vi "Calculate Trapazoidal Profile.vi"(4 "t":dbl, 5 "Max Velocity":dbl, 6 "Final Position":dbl, 7 "Max Acceleration":dbl, 9 "Final Velocity":dbl, 10 "Initial Position":dbl, 11 "Initial Velocity":dbl) -> (2 "Result Position":dbl, 3 "Result Velocity":dbl)   [LabVIEW 2019]
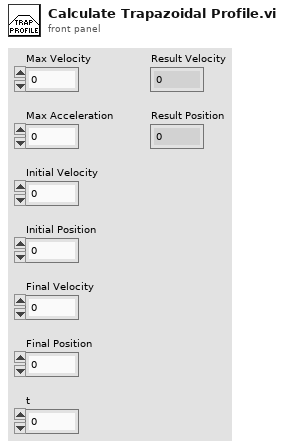
[diagram p1: front panel]
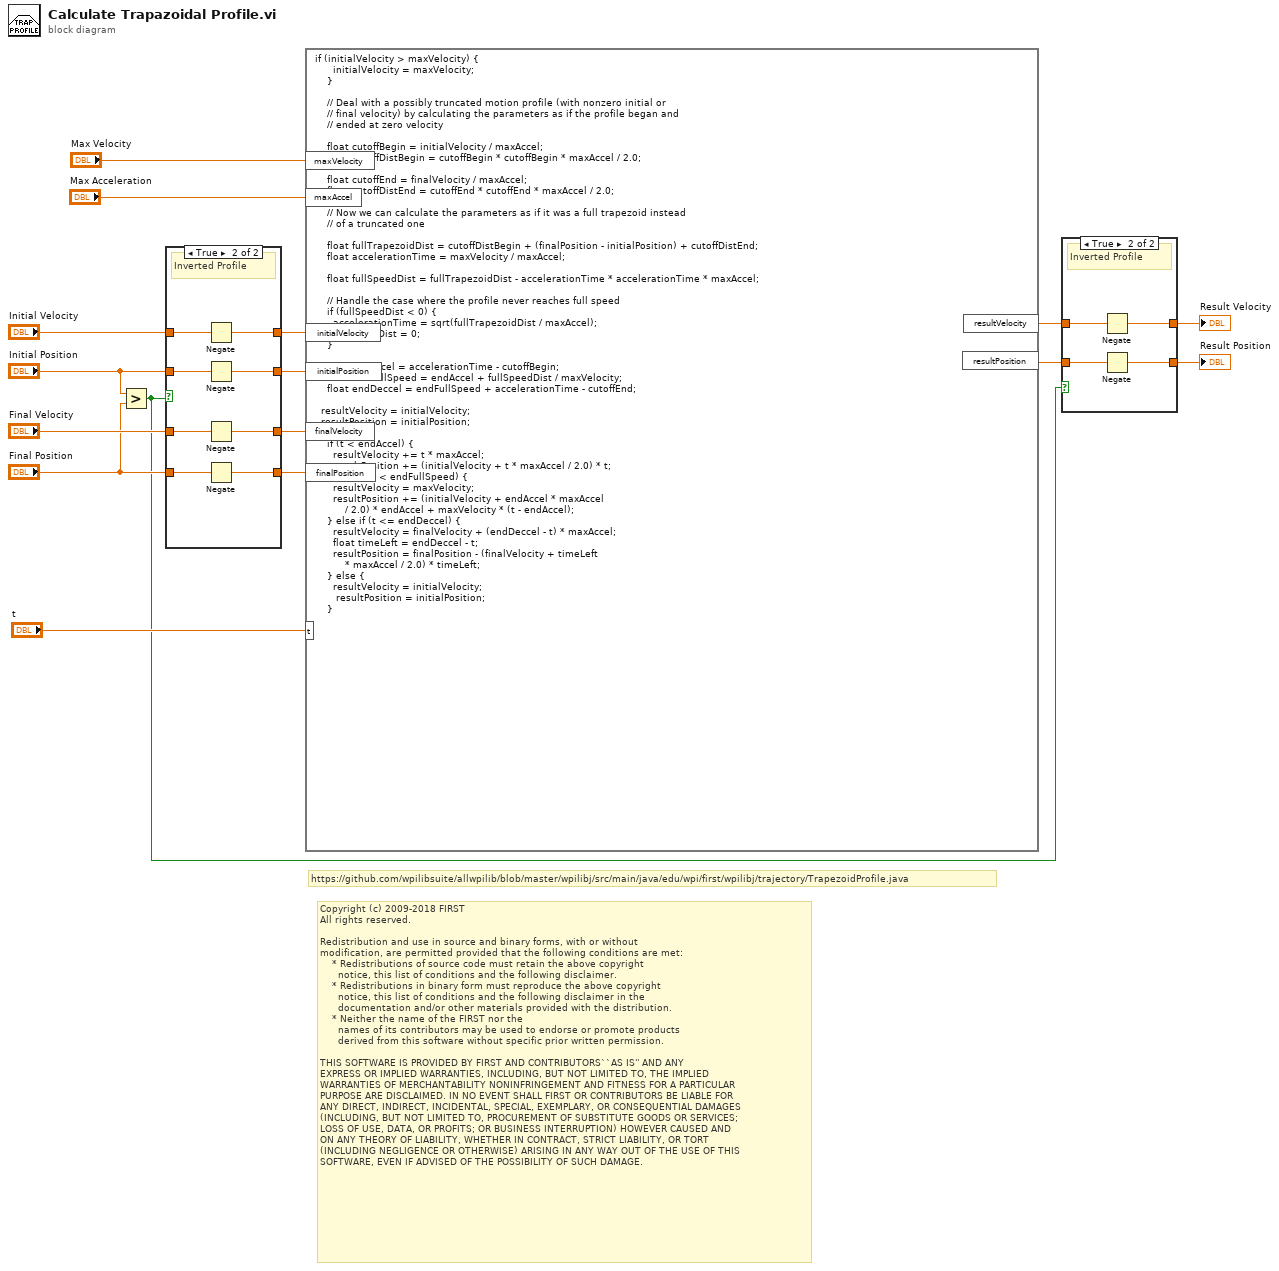
[diagram p0: block diagram]
diagram:
  # "Copyright (c) 2009-2018 FIRST\nAll rights reserved.\n\nRedistribution and use in source and binary forms, with or without\nmodification, are permitted provided that the following conditions are met:\n    * Redistributions of source code must retain the above copyright\n      notice, this list of conditions and the following disclaimer.\n    * Redistributions in binary form must reproduce the above copyright\n      notice, this list of conditions and the following disclaimer in the\n      documentation and/or other materials provided with the distribution.\n    * Neither the name of the FIRST nor the\n      names of its contributors may be used to endorse or promote products\n      derived from this software without specific prior written permission.\n\nTHIS SOFTWARE IS PROVIDED BY FIRST AND CONTRIBUTORS``AS IS'' AND ANY\nEXPRESS OR IMPLIED WARRANTIES, INCLUDING, BUT NOT LIMITED TO, THE IMPLIED\nWARRANTIES OF MERCHANTABILITY NONINFRINGEMENT AND FITNESS FOR A PARTICULAR\nPURPOSE ARE DISCLAIMED. IN NO EVENT SHALL FIRST OR CONTRIBUTORS BE LIABLE FOR\nANY DIRECT, INDIRECT, INCIDENTAL, SPECIAL, EXEMPLARY, OR CONSEQUENTIAL DAMAGES\n(INCLUDING, BUT NOT LIMITED TO, PROCUREMENT OF SUBSTITUTE GOODS OR SERVICES;\nLOSS OF USE, DATA, OR PROFITS; OR BUSINESS INTERRUPTION) HOWEVER CAUSED AND\nON ANY THEORY OF LIABILITY, WHETHER IN CONTRACT, STRICT LIABILITY, OR TORT\n(INCLUDING NEGLIGENCE OR OTHERWISE) ARISING IN ANY WAY OUT OF THE USE OF THIS\nSOFTWARE, EVEN IF ADVISED OF THE POSSIBILITY OF SUCH DAMAGE."
  # "https://github.com/wpilibsuite/allwpilib/blob/master/wpilibj/src/main/java/edu/wpi/first/wpilibj/trajectory/TrapezoidProfile.java"
  n1 = Greater?(x="Initial Position", y="Final Position") -> (0:w1:bool)
  n2 = case shown="True" w1 {
    tunnel: "Final Velocity" -> [w18 w28]
    tunnel: [w18 w27] -> w12
    tunnel: "Final Position" -> [w17 w26]
    tunnel: [w17 w25] -> w10
    tunnel: "Initial Position" -> [w19 w24]
    tunnel: [w19 w23] -> w8
    tunnel: "Initial Velocity" -> [w20 w22]
    tunnel: [w20 w21] -> w6
    frame False {
    }
    frame True {
      # "Inverted Profile"
      n3 = Negate(x=w22) -> (-x=w21:dbl)
      n4 = Negate(x=w24) -> (-x=w23:dbl)
      n5 = Negate(x=w28) -> (-x=w27:dbl)
      n6 = Negate(x=w26) -> (-x=w25:dbl)
    }
  }
  n7 = formula code="if (initialVelocity > maxVelocity) {\n      initialVelocity = maxVelocity;\n    }\n\n    // Deal with a possibly truncated motion profile (with nonzero initial or\n    // final velocity) by calculating the parameters as if the profile began and\n    // ended at zero velocity\n\n    float cutoffBegin = initialVelocity / maxAccel;\n    float cutoffDistBegin = cutoffBegin * cutoffBegin * maxAccel / 2.0;\n\n    float cutoffEnd = finalVelocity / maxAccel;\n    float cutoffDistEnd = cutoffEnd * cutoffEnd * maxAccel / 2.0;\n\n    // Now we can calculate the parameters as if it was a full trapezoid instead\n    // of a truncated one\n\n    float fullTrapezoidDist = cutoffDistBegin + (finalPosition - initialPosition) + cutoffDistEnd;\n    float accelerationTime = maxVelocity / maxAccel;\n\n    float fullSpeedDist = fullTrapezoidDist - accelerationTime * accelerationTime * maxAccel;\n\n    // Handle the case where the profile never reaches full speed\n    if (fullSpeedDist < 0) {\n      accelerationTime = sqrt(fullTrapezoidDist / maxAccel);\n      fullSpeedDist = 0;\n    }\n\n    float endAccel = accelerationTime - cutoffBegin;\n    float endFullSpeed = endAccel + fullSpeedDist / maxVelocity;\n    float endDeccel = endFullSpeed + accelerationTime - cutoffEnd;\n\n  resultVelocity = initialVelocity;\n  resultPosition = initialPosition;\n\n    if (t < endAccel) {\n      resultVelocity += t * maxAccel;\n      resultPosition += (initialVelocity + t * maxAccel / 2.0) * t;\n    } else if (t < endFullSpeed) {\n      resultVelocity = maxVelocity;\n      resultPosition += (initialVelocity + endAccel * maxAccel\n          / 2.0) * endAccel + maxVelocity * (t - endAccel);\n    } else if (t <= endDeccel) {\n      resultVelocity = finalVelocity + (endDeccel - t) * maxAccel;\n      float timeLeft = endDeccel - t;\n      resultPosition = finalPosition - (finalVelocity + timeLeft\n          * maxAccel / 2.0) * timeLeft;\n    } else {\n      resultVelocity = initialVelocity;\n       resultPosition = initialPosition;\n    }"("maxVelocity"="Max Velocity", "maxAccel"="Max Acceleration", "initialVelocity"=w6, "initialPosition"=w8, "finalVelocity"=w12, "finalPosition"=w10, "t"="t") -> ("resultVelocity"=w5:dbl, "resultPosition"=w4:dbl)
  n8 = case shown="True" w1 {
    tunnel: w4 -> [w29 w34]
    tunnel: [w29 w33] -> w3
    tunnel: w5 -> [w30 w32]
    tunnel: [w30 w31] -> w2
    frame False {
    }
    frame True {
      # "Inverted Profile"
      n9 = Negate(x=w32) -> (-x=w31:dbl)
      n10 = Negate(x=w34) -> (-x=w33:dbl)
    }
  }
  "Result Velocity" <- w2
  "Result Position" <- w3
